vi "Run State Update.vi"(11 "Worker Block In":T1={"Block Status"=refnum, "Command Queue"=refnum, "Status"={"Block Status"={"State"=enum."Init", "Next State"=enum."Idle", "Runs"=0, "i"=0, "Init"=FALSE, "Started"=FALSE, "Closing"=FALSE, "Step"=FALSE, "Phase"=enum."N/A", "Worker"=""}, "Error"={"status"=FALSE, "code"=0, "source"=""}}}) -> (3 "Worker Block":T1={"Block Status"=refnum, "Command Queue"=refnum, "Status"={"Block Status"={"State"=enum."Init", "Next State"=enum."Idle", "Runs"=0, "i"=0, "Init"=FALSE, "Started"=FALSE, "Closing"=FALSE, "Step"=FALSE, "Phase"=enum."N/A", "Worker"=""}, "Error"={"status"=FALSE, "code"=0, "source"=""}}})   [LabVIEW 2022 SP3, in "FlexBlocks Support.lvlib"]
uses:
  FlexBlocks Support.lvlib
  Worker Block.ctl
  Block Status with Error.ctl
  Block Status.ctl
  Block State.ctl
  Block Phase.ctl
  Block Command.ctl
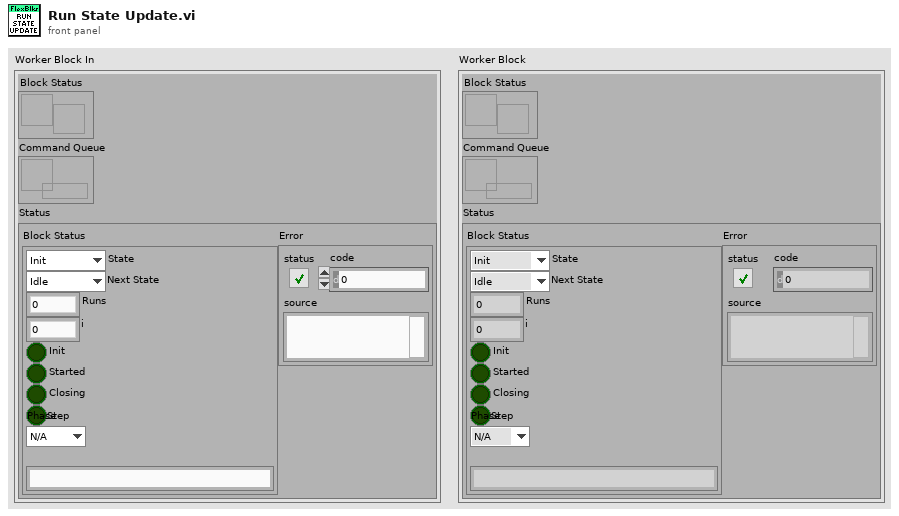
[diagram p1: front panel]
types:
  T1 = typedef "FlexBlocks Support.lvlib/Worker Block.ctl" = cluster{"Block Status":refnum<user-event>, "Command Queue":refnum<queue>, "Status":T2}
  T2 = typedef "FlexBlocks Support.lvlib/Block Status with Error.ctl" = cluster{"Block Status":T3, "Error":errorcluster}
  T3 = typedef "FlexBlocks Support.lvlib/Block Status.ctl" = cluster{"State":T4, "Next State":T4, "Runs":u32, "i":i32, "Init":bool, "Started":bool, "Closing":bool, "Step":bool, "Phase":T5, "Worker":string}
  T4 = typedef "FlexBlocks Support.lvlib/Block State.ctl" = enum16{"Idle", "Init", "Start", "Run", "Stop", "Close"}
  T5 = typedef "FlexBlocks Support.lvlib/Block Phase.ctl" = enum16{"N/A", "Read", "Work", "Write"}
  T6 = typedef "FlexBlocks Support.lvlib/Block Command.ctl" = enum16{"Close", "Init", "Step", "Run", "Pause"}
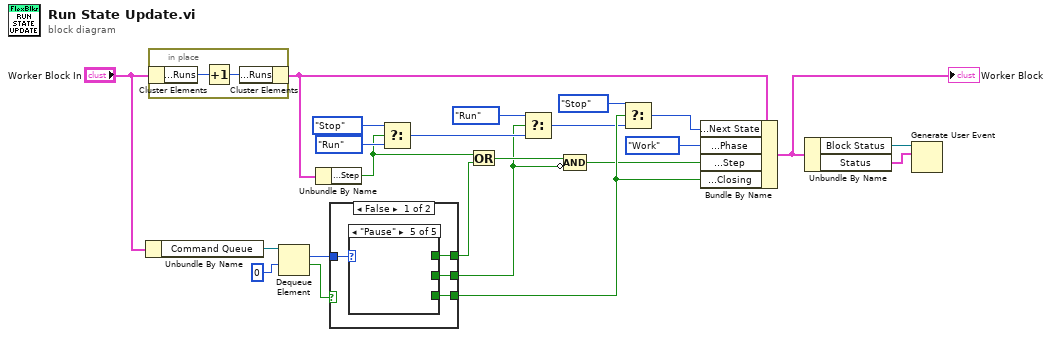
[diagram p0: block diagram]
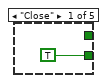
[diagram p2: hidden frame]
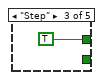
[diagram p4: hidden frame]
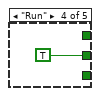
[diagram p5: hidden frame]
diagram:
  n1 = Unbundle By Name("Worker Block In") -> ("Command Queue"=w15:refnum<queue>)
  n2 = in-place {
    n3 = in-place-cluster #1("Worker Block In") -> ("Status.Block Status.Runs"=w25:u32)
    n4 = Increment(x=w25) -> (x+1=w24:u32)
    n5 = in-place-cluster #1("Status.Block Status.Runs"=w24) -> (w19:T1)
  }
  n6 = Dequeue Element(queue=w15, timeout in ms (-1)=0) -> (element=w12:T6, timed out?=w13:bool)  [unwired: 1 in, 2 out]
  n7 = Unbundle By Name(w19) -> ("Status.Block Status.Step"=w7:bool)
  n8 = case shown="False" w13 {
    tunnel: w12 -> [w29 _]
    tunnel: [w28 _] -> w9
    tunnel: [w27 _] -> w6
    tunnel: [w26 _] -> w1
    frame False {
      n9 = case shown="\"Pause\"" w29 {
        tunnel: [TRUE _ _ _ _] -> w28
        tunnel: [_ _ TRUE _ _] -> w27
        tunnel: [_ _ _ TRUE _] -> w26
        frame "Close" {
        }
        frame "Init" {
        }
        frame "Step" {
        }
        frame "Run" {
        }
        frame "Pause" {
        }
      }
    }
    frame True {
    }
  }
  n10 = Select(t=Block_State."Stop" ("Status.Block Status.Next State"), s=w7, f=Block_State."Run" ("Status.Block Status.Next State")) -> (s? t:f=w4:T4)
  n11 = Or(x=w7, y=w6) -> (x .or. y?=w8:bool)
  n12 = Select(t=Block_State."Run", s=w1, f=w4) -> (s? t:f=w3:T4)
  n13 = Compound Arithmetic op=AND(w8, invert w1) -> (w5:bool)
  n14 = Select(t=Block_State."Stop", s=w9, f=w3) -> (s? t:f=w11:T4)
  n15 = Bundle By Name(cluster=w19, "Status.Block Status.Next State"=w11, "Status.Block Status.Phase"=Block_Phase."Work", "Status.Block Status.Step"=w5, "Status.Block Status.Closing"=w9) -> (w22:T1)
  "Worker Block" <- w22
  n16 = Unbundle By Name(w22) -> ("Block Status"=w21:refnum<user-event>, "Status"=w20:T2)
  n17 = Generate User Event(user event=w21, event data cluster=w20) -> ()  [unwired: 2 in, 2 out]
